vi "Calibrar.vi"() -> ()   [LabVIEW 2017]
panel:
  out "Numeric":dbl
  in  "Calibrar":bool
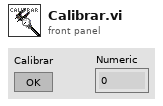
[diagram p1: front panel]
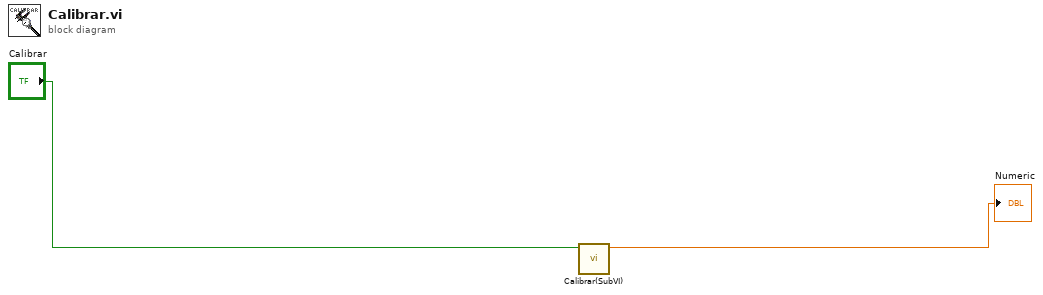
[diagram p0: block diagram]
diagram:
  n1 = call "Calibrar(SubVI).vi"("Calibrar"="Calibrar") -> ("Relación"=→"Numeric":dbl)  [unwired: 10 in]
